vi "Velocity.vi"() -> (1 "VZ":dbl, 2 "VY":dbl, 3 "VX":dbl)   [LabVIEW 2017]
uses:
  <userlib>/HapticSTM/Feedbackless - Testdata/Project/feedbackless.lvproj/feedbackless.lvproj/C/Program Files/National Instruments/LabVIEW 2019/user.lib/HapticSTM/HapticSTM.lvlib
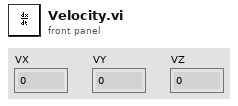
[diagram p1: front panel]
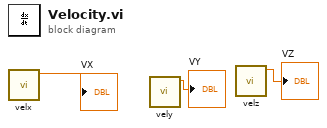
[diagram p0: block diagram]
diagram:
  n1 = call <userlib>:"velx.vi"() -> ("function return"=→"VX":dbl)  [unwired: 11 in]
  n2 = call <userlib>:"vely.vi"() -> ("function return"=→"VY":dbl)  [unwired: 11 in]
  n3 = call <userlib>:"velz.vi"() -> ("function return"=→"VZ":dbl)  [unwired: 11 in]
